vi "纳清_第三点校准数据写入.vi"(7 "探头":T1(ring), 8 "error in (no error)":errorcluster caption="错误输入（无错误）", 10 "数值":sgl, 11 "MB session in":refnum<class "MB_Master.lvclass">) -> (0 "error out":errorcluster caption="错误输出", 3 "MB session out":refnum<class "MB_Master.lvclass">)   [LabVIEW 2016, in "斯坦道多参数.lvlib"]
uses:
  <vilib>/Plasmionique/MB Master/MB Master.lvlib
  <vilib>/Plasmionique/MB Master/MB_Master/MB_Master.lvclass
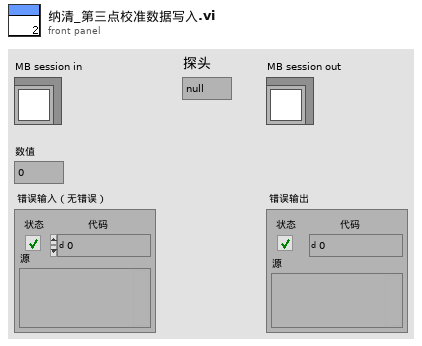
[diagram p1: front panel]
types:
  T1 = enum16{"null", "pH", "DO", "浊度", "电导率", "叶绿素a", "藻密度", "氨氮"}
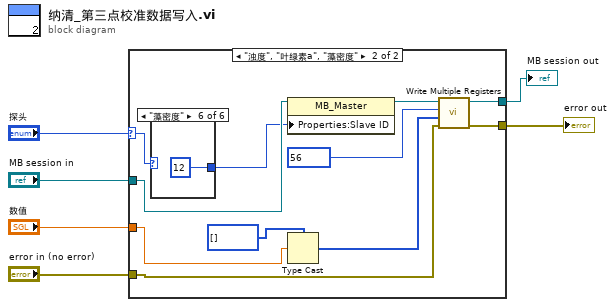
[diagram p0: block diagram]
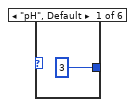
[diagram p3: hidden frame]
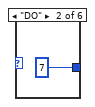
[diagram p4: hidden frame]
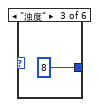
[diagram p5: hidden frame]
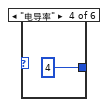
[diagram p6: hidden frame]
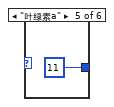
[diagram p7: hidden frame]
diagram:
  n1 = case shown="\"浊度\", \"叶绿素a\", \"藻密度\"" "探头" {
    selector: "探头" -> [_ w19]
    tunnel: "MB session in" -> [w8 w14]
    tunnel: [w8 w13] -> w4
    tunnel: [w7 w12] -> w3
    tunnel: "error in (no error)" -> [w7 w11]
    tunnel: "数值" -> [_ w10]
    frame "pH", Default {
    }
    frame "浊度", "叶绿素a", "藻密度" {
      n2 = case shown="\"藻密度\"" w19 {
        tunnel: [3 7 8 4 11 12] -> w9
        frame "pH", Default {
        }
        frame "DO" {
        }
        frame "浊度" {
        }
        frame "电导率" {
        }
        frame "叶绿素a" {
        }
        frame "藻密度" {
        }
      }
      n3 = property class="MB_Master"(reference=w14, "Properties:Slave ID"=w9) -> (reference out=w16:refnum<class "MB_Master.lvclass">)  [unwired: 1 in, 1 out]
      n4 = Type Cast(type=u16[] [], x=w10) -> (*(type *) &x=w18:u16[])
      n5 = call <vilib>:"Write Multiple Registers.vi"("error in (no error)"=w11, "values"=w18, "starting address"=u16 56, "MB session in"=w16) -> ("error out"=w12:errorcluster, "MB session out"=w13:refnum<class "MB_Master.lvclass">)  [unwired: 6 in]
    }
  }
  "MB session out" <- w4
  "error out" <- w3
